vi "Reverse_filepath.vi"(1 "Filename":path) -> (0 "Reversed Filepath":string)   [LabVIEW 2010]
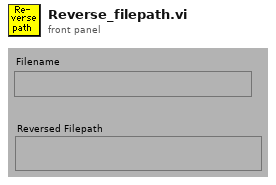
[diagram p1: front panel]
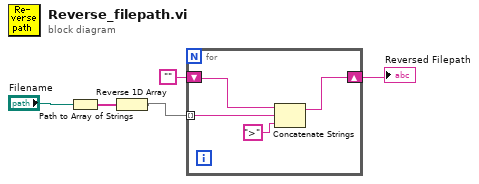
[diagram p0: block diagram]
diagram:
  n1 = Path to Array of Strings(0:"Filename") -> (2:w5:string[])  [unwired: 1 out]
  n2 = Reverse 1D Array(array=w5) -> (reversed array=w4:string[])
  n3 = for {
    shift-right: [w8] -> w3
    shift-left: "" -> [w9]
    tunnel: w4 -> [w7] mode=indexing
    n4 = Concatenate Strings(w9, w7, ">" ("Substring")) -> (w8:string)
  }
  "Reversed Filepath" <- w3
